vi "CPU_Gen_Filter_Coefs.vi"(8 "error in":errorcluster, 11 "FIR Config":T1={"filter type"=enum."Lowpass", "taps"=1024, "high cutoff freq: fh"=0.45, "sampling freq: fs"=40000000.0, "low cutoff freq: fl"=200000.0, "window"=0, "option"=enum."not scaled"} {"window" items=["Rectangle"=0, "Hanning"=1, "Hamming"=2, "Blackman-Harris"=3, "Exact Blackman"=4, "Blackman"=5, "Flat Top"=6, "4 Term B-Harris "=7, "7 Term B-Harris"=8, "Low Sidelobe"=9, "Blackman Nuttall"=11, "Triangle"=30, "Bartlett-Hanning"=31, "Bohman"=32, "Parzen"=33, "Welch"=34, "Kaiser"=60, "Dolph-Chebyshev"=61, "Gaussian"=62]; "low cutoff freq: fl" format="%#_13p"; "sampling freq: fs" format="%#_13p"; "high cutoff freq: fh" format="%#_13g"}) -> (0 "error out":errorcluster, 3 "FIR_Coeffs":dbl[](array[numeric]), 5 "FIR Init/Continue":bool)   [LabVIEW 2020]
uses:
  Controls/FIR_Config.ctl
  <vilib>/Analysis/3filter.llb/Filter Passband Type.ctl
  <vilib>/Analysis/4window.llb/windowTd.ctl
  dcd26b71-38d5-4fa1-bb65-21529362c854.vi
  <vilib>/Analysis/NI_AALBase.lvlib
  <vilib>/Analysis/NI_AALPro.lvlib
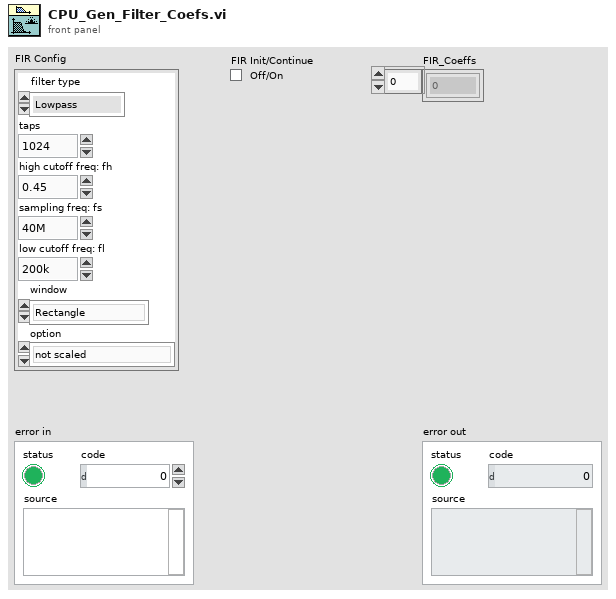
[diagram p1: front panel]
types:
  T1 = typedef "FIR_Config.ctl" = cluster{"filter type":T2, "taps":i32, "high cutoff freq: fh":dbl, "sampling freq: fs":dbl, "low cutoff freq: fl":dbl, "window":T3, "option":enum32{"not scaled", "scaled"}}
  T2 = typedef "NI_AALBase.lvlib/Filter Passband Type.ctl" = enum32{"Lowpass", "Highpass", "Bandpass", "Bandstop"}
  T3 = typedef "NI_AALPro.lvlib/windowTd.ctl" = u32
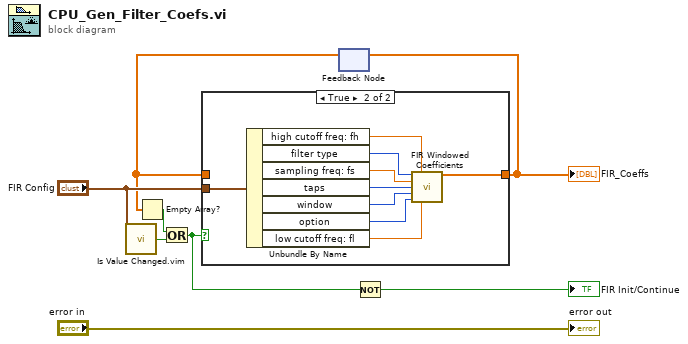
[diagram p0: block diagram]
diagram:
  n1 = call "Is Value Changed.vim"("value"="FIR Config") -> ("changed or first call?"=w6:bool)
  n2 = feedback #1() -> (w4:dbl[])  [unwired: 1 in]
  n3 = Empty Array?(array=w4) -> (empty?=w5:bool)
  n4 = Or(x=w5, y=w6) -> (x .or. y?=w2:bool)
  n5 = case shown="True" w2 {
    tunnel: "FIR Config" -> [_ w18]
    tunnel: [w9 w10] -> w7
    tunnel: w4 -> [w9 _]
    frame False {
    }
    frame True {
      n6 = Unbundle By Name(w18) -> ("high cutoff freq: fh"=w12:dbl, "filter type"=w17:T2, "sampling freq: fs"=w16:dbl, "taps"=w15:i32, "window"=w14:T3, "option"=w13:enum32{"not scaled", "scaled"}, "low cutoff freq: fl"=w11:dbl)
      n7 = call <vilib>:"FIR Windowed Coefficients.vi"("filter type"=w17, "high cutoff freq: fh"=w12, "sampling freq: fs"=w16, "taps"=w15, "window"=w14, "option"=w13, "low cutoff freq: fl"=w11) -> ("FIR Windowed Coefficients"=w10:dbl[])  [unwired: 7 in, 1 out]
    }
  }
  "FIR_Coeffs" <- w7
  n8 = feedback-in #1(w7) -> ()
  n9 = Not(x=w2) -> (.not. x?=→"FIR Init/Continue":bool)
  "error out" <- "error in"
